vi "Display Info.vi"(7 "Layout ref":refnum<vi>, 8 "error in (no error)":errorcluster, 9 "Modify (F) /Add [T]":bool, 10 "Names in use":string[](array[string]), 11 "Agilent ESG in":refnum<class "Agilent ESG.lvclass">) -> (0 "error out":errorcluster, 1 "Names in use out":string[](array[string]), 2 "Changes Made?":bool, 3 "Agilent ESG out":refnum<class "Agilent ESG.lvclass">)   [LabVIEW 2013, in "Agilent ESG.lvclass"]
uses:
  Agilent ESG.lvclass
  TypeDefs/ColumnAppearCluster.ctl
  Agilent ESG.lvclass/Agilent ESG.ctl
  ColumnVIs/Column/Column.lvclass
panel:
  in  "Appearance in Table":T2(array[cluster])=[{"Channel Name"="0", "Columns' Appearance"=[{"Column Name"="", "Width"=30, "Bkgd"=[16448250], "Text"=[0]}, {"Column Name"="", "Width"=30, "Bkgd"=[16448250], "Text"=[0]}, {"Column Name"="", "Width"=30, "Bkgd"=[16448250], "Text"=[0]}]}, {"Channel Name"="1", "Columns' Appearance"=[{"Column Name"="", "Width"=30, "Bkgd"=[16448250], "Text"=[0]}, {"Column Name"="", "Width"=30, "Bkgd"=[16448250], "Text"=[0]}, {"Column Name"="", "Width"=30, "Bkgd"=[16448250], "Text"=[0]}]}, {"Channel Name"="2", "Columns' Appearance"=[{"Column Name"="", "Width"=30, "Bkgd"=[16448250], "Text"=[0]}, {"Column Name"="", "Width"=30, "Bkgd"=[16448250], "Text"=[0]}, {"Column Name"="", "Width"=30, "Bkgd"=[16448250], "Text"=[0]}]}, {"Channel Name"="3", "Columns' Appearance"=[{"Column Name"="", "Width"=30, "Bkgd"=[16448250], "Text"=[0]}, {"Column Name"="", "Width"=30, "Bkgd"=[16448250], "Text"=[0]}, {"Column Name"="", "Width"=30, "Bkgd"=[16448250], "Text"=[0]}]}]
  in  "Hardware Settings":T3={"PB Trigger Line"=4, "Serial Port"=""}
  in  "Name":string
  in  "Device Description":string
  in  "Done":bool
  in  "Cancel":bool
  # "This VI just sets the wiring structure.\nOpen a child override version instead!"
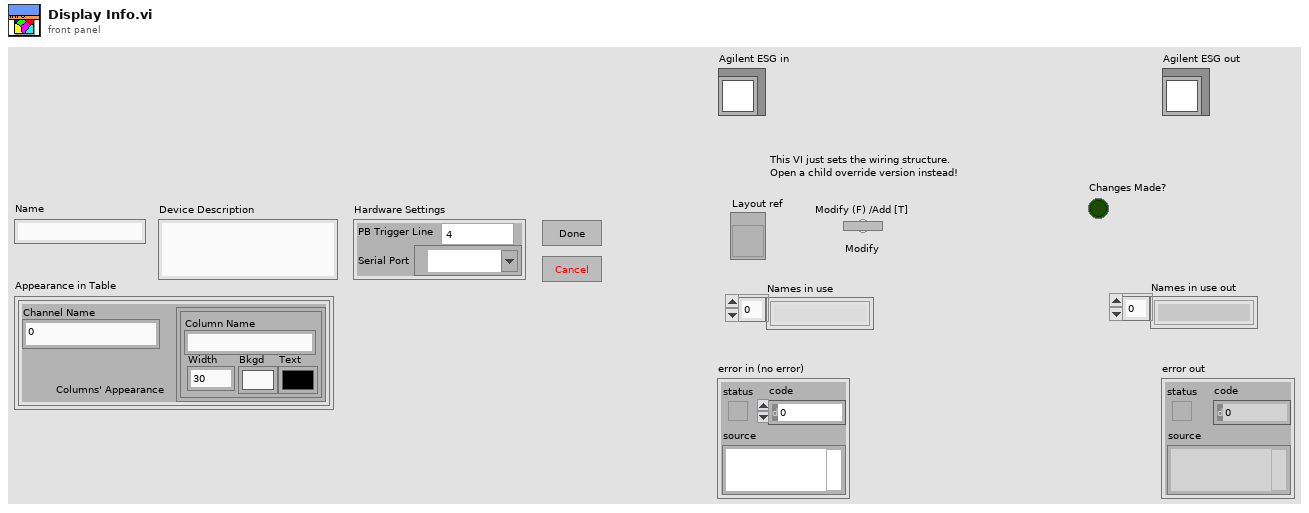
[diagram p1: front panel]
types:
  T1 = typedef "ColumnAppearCluster.ctl" = cluster{"Column Name":string, "Width":u32, "Bkgd":u32[], "Text":u32[]}
  T2 = cluster{"Channel Name":string, "Columns' Appearance":T1[]}[]
  T3 = cluster{"PB Trigger Line":u16, "Serial Port":refnum<visa-resource-name>}
  T4 = cluster{"Channel Name":bool, "Columns' Appearance":cluster{"Column Name":bool, "Width":bool, "Bkgd":bool[], "Text":bool[]}[]}[]
  T5 = cluster{"Channel Name":string, "Columns' Appearance":T1[]}
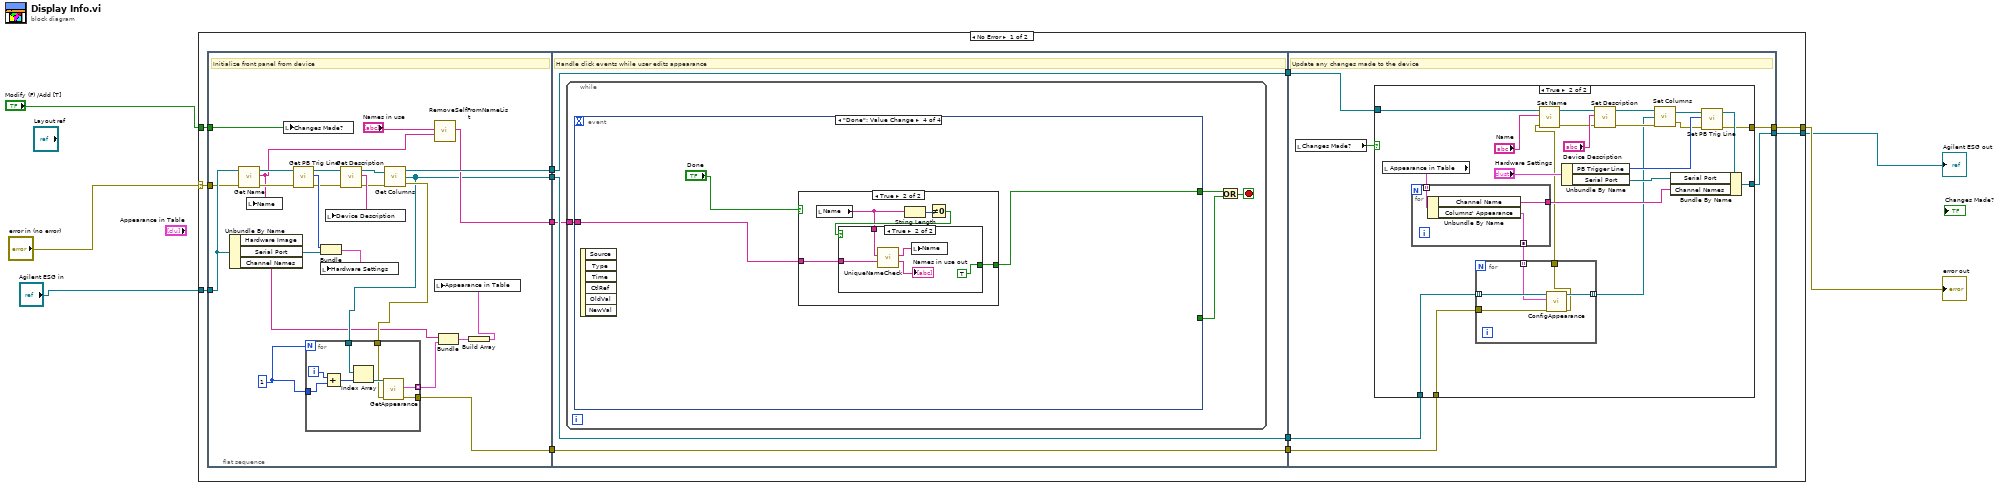
[diagram p0: block diagram]
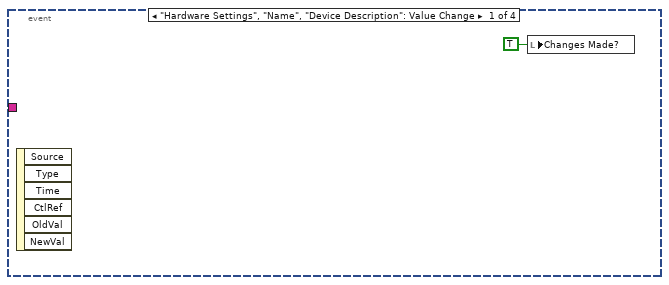
[diagram p2: hidden frame]
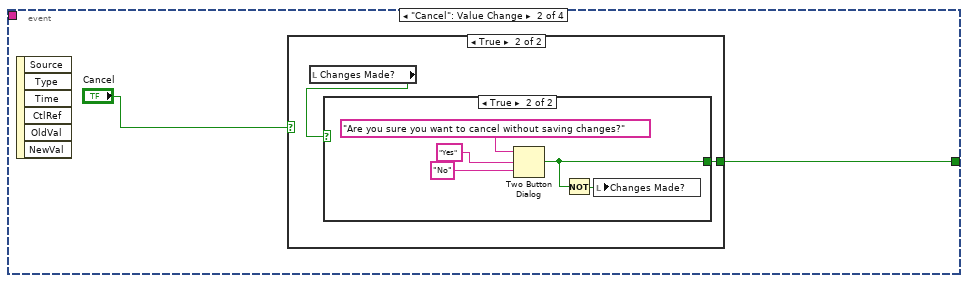
[diagram p3: hidden frame]
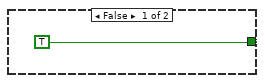
[diagram p5: hidden frame]
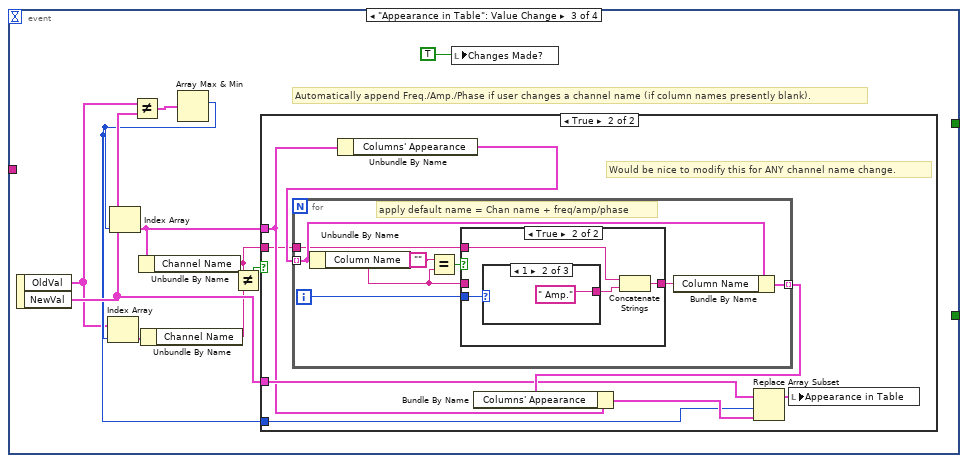
[diagram p6: hidden frame]
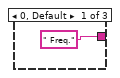
[diagram p9: hidden frame]
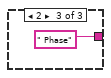
[diagram p10: hidden frame]
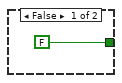
[diagram p11: hidden frame]
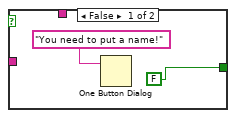
[diagram p12: hidden frame]
diagram:
  n1 = case shown="No Error" "error in (no error)" {
    selector: "error in (no error)" -> [w9 w159]
    tunnel: "Agilent ESG in" -> [w17 w160]
    tunnel: [w16 w160] -> w1
    tunnel: [w8 w159] -> w2
    tunnel: "Modify (F) /Add [T]" -> [w7 _]
    frame No Error {
      n2 = flat-sequence {
        tunnel: w17 -> [w40]
        tunnel: [w34] -> w15
        tunnel: [w21] -> w13
        tunnel: [w23] -> w10
        tunnel: w9 -> [w30]
        tunnel: w7 -> [w29]
        tunnel: [w27] -> w6
        tunnel: w15 -> [w54]
        tunnel: [w54] -> w14
        tunnel: w13 -> [w53]
        tunnel: [w53] -> w12
        tunnel: [w52] -> w11
        tunnel: w10 -> [w52]
        tunnel: w6 -> [w51]
        tunnel: [w126] -> w16
        tunnel: w14 -> [w125]
        tunnel: w12 -> [w123]
        tunnel: w11 -> [w122]
        tunnel: [w121] -> w8
        frame #0 {
          w25 = 1
          # "Initialize front panel from device"
          n3 = Unbundle By Name(w40) -> ("Serial Port"=w42:refnum<visa-resource-name>, "Channel Names"=w20:string)  [unwired: 1 out]
          n4 = call-dynamic "Get Name.vi"("error in (no error)"=w30, "Device in"=w40) -> ("error out"=w33:errorcluster, "Name"=w28:string, "Device out"=w41:refnum<class "Agilent ESG.lvclass">)  [unwired: 7 in]
          n5 = local write "Name"(w28) -> ()
          n6 = local write "Changes Made?"(w29) -> ()
          n7 = call-dynamic "Get PB Trig Line.vi"("error in (no error)"=w33, "Device in"=w41) -> ("error out"=w32:errorcluster, "PB Trigger Line"=w36:u16, "Device out"=w38:refnum<class "Agilent ESG.lvclass">)  [unwired: 7 in]
          n8 = Bundle("PB Trigger Line"=w36, "Serial Port"=w42) -> (w37:T3)  [unwired: 1 in]
          n9 = local write "Hardware Settings"(w37) -> ()
          n10 = call-dynamic "Get Description.vi"("error in (no error)"=w32, "Device in"=w38) -> ("error out"=w31:errorcluster, "Device Description"=w39:string, "Device out"=w35:refnum<class "Agilent ESG.lvclass">)  [unwired: 7 in]
          n11 = local write "Device Description"(w39) -> ()
          n12 = call-dynamic "Get Columns.vi"("Device in"=w35, "error in (no error)"=w31) -> ("Device out"=w34:refnum<class "Agilent ESG.lvclass">, "Columns"=w21:refnum<class "Column.lvclass">[], "error out"=w22:errorcluster)
          n13 = for {
            N: w25 -> [_]
            tunnel: w21 -> [w50]
            tunnel: w25 -> [w47]
            tunnel: w22 -> [w45]
            tunnel: [w44] -> w24 mode=indexing
            tunnel: [w43] -> w23
            i -> [w46]
            n14 = Add(x=w46, y=w47) -> (x+y=w49:i32)
            n15 = Index Array(array=w50, index=w49) -> (element=w48:refnum<class "Column.lvclass">)
            n16 = call "GetAppearance.vi"("error in (no error)"=w45, "Column in"=w48) -> ("error out"=w43:errorcluster, "Column Appearance"=w44:T1)  [unwired: 7 in, 1 out]
          }
          n17 = call "RemoveSelfFromNameList.vi"("self Name"=w28, "Names in use"="Names in use") -> ("Reserved Names"=w27:string[])  [unwired: 9 in]
          n18 = Bundle("Channel Names"=w20, w24) -> (w19:cluster{"Channel Names":string, T1[]})  [unwired: 1 in]
          n19 = Build Array(w19) -> (w18:cluster{"Channel Names":string, T1[]}[])
          n20 = local write "Appearance in Table"(w18) -> ()
        }
        frame #1 {
          # "Handle click events while user edits appearance"
          n21 = while {
            tunnel: w51 -> [w55]
            stop <- w58 stop-if-true
            n22 = event shown="[3] \"Done\": Value Change" {
              selector: _ -> [_ _ _ _]
              dyn-events: _ -> [_ _ _ _]
              timeout: _ -> [_ _ _ _]
              tunnel: [_ w60 _ _] -> w57
              tunnel: [_ _ _ w106] -> w56
              tunnel: w55 -> [_ _ _ w105]
              event "Hardware Settings", "Name", "Device Description": Value Change {
                n23 = event-data() -> ()  [unwired: 1 in, 6 out]
                n24 = local write "Changes Made?"(TRUE ("Changes Made?")) -> ()
              }
              event "Cancel": Value Change {
                n25 = event-data() -> ()  [unwired: 1 in, 6 out]
                n26 = case shown="True" "Cancel" {
                  selector: "Cancel" -> [w62 _]
                  tunnel: [w62 w64] -> w60
                  frame False {
                  }
                  frame True {
                    n27 = local read "Changes Made?"() -> (w63:bool)
                    n28 = case shown="True" w63 {
                      tunnel: [TRUE w67] -> w64
                      frame False {
                      }
                      frame True {
                        n29 = Two Button Dialog(message="Are you sure you want to cancel without saving changes?", 1:"No", 2:"Yes") -> (T button?=w67:bool)
                        n30 = Not(x=w67) -> (.not. x?=w66:bool)
                        n31 = local write "Changes Made?"(w66) -> ()
                      }
                    }
                  }
                }
              }
              event "Appearance in Table": Value Change {
                # "Automatically append Freq./Amp./Phase if user changes a channel name (if column names presently blank)."
                n32 = event-data() -> ("OldVal"=w76:T2, "NewVal"=w78:T2)  [unwired: 1 in]
                n33 = Not Equal?(x=w76, y=w78) -> (x != y?=w79:T4)
                n34 = Array Max & Min(array=w79) -> (max index (indices)=w77:i32)  [unwired: 3 out]
                n35 = Index Array(array=w76, index=w77) -> (element=w75:T5)
                n36 = Index Array(array=w78, index=w77) -> (element=w74:T5)
                n37 = Unbundle By Name(w74) -> ("Channel Name"=w73:string)
                n38 = Unbundle By Name(w75) -> ("Channel Name"=w72:string)
                n39 = Not Equal?(x=w73, y=w72) -> (x != y?=w71:bool)
                n40 = case shown="True" w71 {
                  tunnel: w78 -> [_ w85]
                  tunnel: w77 -> [_ w83]
                  tunnel: w74 -> [_ w82]
                  tunnel: w73 -> [_ w81]
                  frame False {
                  }
                  frame True {
                    # "Would be nice to modify this for ANY channel name change."
                    n41 = Unbundle By Name(w82) -> ("Columns' Appearance"=w88:T1[])
                    n42 = for {
                      tunnel: w88 -> [w92] mode=indexing
                      tunnel: [w93] -> w87 mode=indexing
                      tunnel: w81 -> [w91]
                      i -> [w95]
                      # "apply default name = Chan name + freq/amp/phase"
                      n43 = Unbundle By Name(w92) -> ("Column Name"=w89:string)
                      n44 = Equal?(x="", y=w89) -> (x = y?=w94:bool)
                      n45 = case shown="True" w94 {
                        tunnel: [w97 w99] -> w96
                        tunnel: w95 -> [_ w101]
                        tunnel: w91 -> [_ w98]
                        tunnel: w89 -> [w97 _]
                        frame False {
                        }
                        frame True {
                          n46 = case shown="1" w101 {
                            tunnel: [" Freq." " Amp." " Phase"] -> w100
                            frame 0, Default {
                            }
                            frame 1 {
                            }
                            frame 2 {
                            }
                          }
                          n47 = Concatenate Strings(w98, w100) -> (w99:string)
                        }
                      }
                      n48 = Bundle By Name(cluster=w92, "Column Name"=w96) -> (w93:T1)
                    }
                    n49 = Bundle By Name(cluster=w82, "Columns' Appearance"=w87) -> (w86:T5)
                    n50 = Replace Array Subset(array=w85, new element=w86, index=w83) -> (w84:T2)
                    n51 = local write "Appearance in Table"(w84) -> ()
                  }
                }
                n52 = local write "Changes Made?"(TRUE) -> ()
              }
              event "Done": Value Change {
                n53 = event-data() -> ()  [unwired: 1 in, 6 out]
                n54 = case shown="True" "Done" {
                  tunnel: [FALSE w111] -> w106
                  tunnel: w105 -> [_ w109]
                  frame False {
                  }
                  frame True {
                    n55 = local read "Name"() -> (w110:string)
                    n56 = String Length(string=w110) -> (length=w113:i32)
                    n57 = Not Equal To 0?(x=w113) -> (x != 0?=w112:bool)
                    n58 = case shown="True" w112 {
                      tunnel: [FALSE TRUE] -> w111
                      tunnel: w110 -> [_ w119]
                      tunnel: w109 -> [_ w117]
                      frame False {
                        n59 = One Button Dialog(message="You need to put a name!") -> ()  [unwired: 1 in, 1 out]
                      }
                      frame True {
                        n60 = call "UniqueNameCheck.vi"("Names in use"=w117, "Device Name"=w119) -> ("Names in use out"=→"Names in use out":string[], "Unique name"=w118:string)  [unwired: 8 in]
                        n61 = local write "Name"(w118) -> ()
                      }
                    }
                  }
                }
              }
            }
            n62 = Or(x=w56, y=w57) -> (x .or. y?=w58:bool)
          }
        }
        frame #2 {
          # "Update any changes made to the device"
          n63 = local read "Changes Made?"() -> (w124:bool)
          n64 = case shown="True" w124 {
            tunnel: [w128 w150] -> w126
            tunnel: w125 -> [w128 w145]
            tunnel: w123 -> [_ w134]
            tunnel: w122 -> [w127 w132]
            tunnel: [w127 w130] -> w121
            frame False {
            }
            frame True {
              n65 = local read "Appearance in Table"() -> (w135:T2)
              n66 = for {
                tunnel: [w158] -> w149
                tunnel: w135 -> [w157] mode=indexing
                tunnel: [w156] -> w133 mode=concatenating
                n67 = Unbundle By Name(w157) -> ("Channel Name"=w158:string, "Columns' Appearance"=w156:T1[])
              }
              n68 = for {
                tunnel: w134 -> [w155] mode=indexing
                tunnel: w133 -> [w154] mode=indexing
                tunnel: w132 -> [w153]
                tunnel: [w152] -> w131 mode=indexing
                tunnel: [w151] -> w129
                n69 = call "ConfigAppearance.vi"("error in (no error)"=w153, "Column Appearance"=w154, "Column in"=w155) -> ("error out"=w151:errorcluster, "Column out"=w152:refnum<class "Column.lvclass">)  [unwired: 7 in]
              }
              n70 = call-dynamic "Set Name.vi"("error in (no error)"=w129, "Name"="Name", "Device in"=w145) -> ("error out"=w137:errorcluster, "Device out"=w147:refnum<class "Agilent ESG.lvclass">)  [unwired: 7 in]
              n71 = Unbundle By Name("Hardware Settings") -> ("PB Trigger Line"=w140:u16, "Serial Port"=w142:refnum<visa-resource-name>)
              n72 = call-dynamic "Set Description.vi"("error in (no error)"=w137, "Device Description"="Device Description", "Device in"=w147) -> ("error out"=w136:errorcluster, "Device out"=w146:refnum<class "Agilent ESG.lvclass">)  [unwired: 7 in]
              n73 = call-dynamic "Set Columns.vi"("error in (no error)"=w136, "Columns"=w131, "Device in"=w146) -> ("error out"=w138:errorcluster, "Device out"=w139:refnum<class "Agilent ESG.lvclass">)  [unwired: 1 in]
              n74 = call-dynamic "Set PB Trig Line.vi"("error in (no error)"=w138, "PB Trigger Line"=w140, "Device in"=w139) -> ("error out"=w130:errorcluster, "Device out"=w141:refnum<class "Agilent ESG.lvclass">)  [unwired: 7 in]
              n75 = Bundle By Name(cluster=w141, "Serial Port"=w142, "Channel Names"=w149) -> (w150:refnum<class "Agilent ESG.lvclass">)
            }
          }
        }
      }
    }
    frame Error {
    }
  }
  "error out" <- w2
  "Agilent ESG out" <- w1
